vi "Apply Endpoint.vi"(10 "Endpoint Config":T3[](array[typedef]), 11 "Destination In":T2) -> (1 "Have audiogram":bool, 2 "Modality":T1, 3 "Destination Out":T2)   [LabVIEW 2020, in "Stimulus Channel (G3).xctl"]
uses:
  Stimulus Channel (G3).xctl
  Typedefs/Destination.ctl
  Calibration VIs/Endpoint VIs/LV Source/Endpoint-Spec.ctl
  Calibration VIs/Endpoint VIs/LV Source/Endpoint-Modality.ctl
  Calibration VIs/Endpoint VIs/LV Source/Endpoint-Laterality.ctl
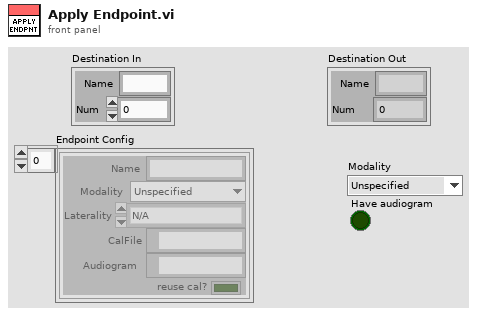
[diagram p1: front panel]
types:
  T1 = typedef "Endpoint-Modality.ctl" = enum16{"Unspecified", "Acoustic", "Electric", "Optical"}
  T2 = typedef "Destination.ctl" = cluster{"Name":string, "Num":i32}
  T3 = typedef "Endpoint-Spec.ctl" = cluster{"Name":string, "Modality":T1, "Laterality":T4, "CalFile":path, "Audiogram":path, "reuse cal?":bool}
  T4 = typedef "Endpoint-Laterality.ctl" = enum16{"N/A", "Right", "Left"}
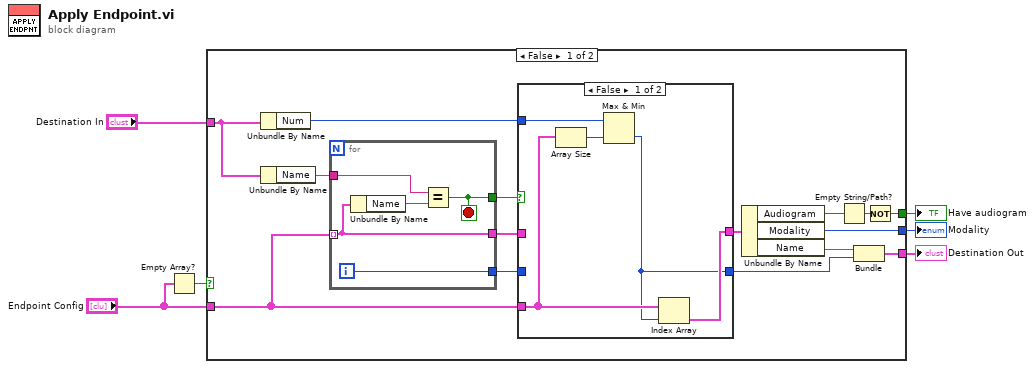
[diagram p0: block diagram]
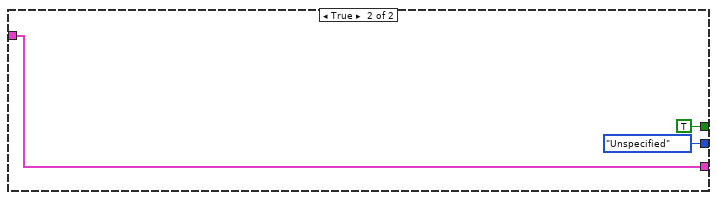
[diagram p3: hidden frame]
diagram:
  n1 = Empty Array?(array="Endpoint Config") -> (empty?=w5:bool)
  n2 = case shown="False" w5 {
    tunnel: "Endpoint Config" -> [w15 _]
    tunnel: "Destination In" -> [w18 w34]
    tunnel: [w11 w34] -> w3
    tunnel: [w10 Endpoint-Modality."Unspecified" ("Modality")] -> w2
    tunnel: [w7 TRUE] -> w1
    frame False {
      n3 = Unbundle By Name(w18) -> ("Num"=w16:i32)
      n4 = Unbundle By Name(w18) -> ("Name"=w21:string)
      n5 = for {
        tunnel: w15 -> [w30] mode=indexing
        tunnel: w21 -> [w32]
        tunnel: [w31] -> w19
        tunnel: [w30] -> w20
        tunnel: [w29] -> w17
        i -> [w29]
        stop <- w31 stop-if-true
        n6 = Unbundle By Name(w30) -> ("Name"=w33:string)
        n7 = Equal?(x=w32, y=w33) -> (x = y?=w31:bool)
      }
      n8 = case shown="False" w19 {
        tunnel: w20 -> [_ w28]
        tunnel: [w23 w28] -> w14
        tunnel: w17 -> [_ w27]
        tunnel: w16 -> [w26 _]
        tunnel: w15 -> [w24 _]
        tunnel: [w22 w27] -> w12
        frame False {
          n9 = Array Size(array=w24) -> (size(s)=w25:i32)
          n10 = Max & Min(x=w26, y=w25) -> (min(x,y)=w22:i32)  [unwired: 1 out]
          n11 = Index Array(array=w24, index=w22) -> (element=w23:T3)
        }
        frame True {
        }
      }
      n12 = Unbundle By Name(w14) -> ("Audiogram"=w9:path, "Modality"=w10:T1, "Name"=w13:string)
      n13 = Empty String/Path?(string/path=w9) -> (empty?=w8:bool)
      n14 = Bundle("Name"=w13, w12) -> (w11:cluster{"Name":string, i32})  [unwired: 1 in]
      n15 = Not(x=w8) -> (.not. x?=w7:bool)
    }
    frame True {
    }
  }
  "Destination Out" <- w3
  "Modality" <- w2
  "Have audiogram" <- w1
